vi "Measurement Parser.vi"(8 "error in (no error)":errorcluster, 10 "Data Array":dbl[](array[numeric]), 11 "Yokogawa WT2X0 in":refnum<class "Yokogawa WT2X0.lvclass">) -> (0 "error out":errorcluster, 2 "output cluster":T1, 3 "Yokogawa WT2X0 out":refnum<class "Yokogawa WT2X0.lvclass">)   [LabVIEW 2012, in "Universal Power Meter.lvlib" / "Yokogawa WT2X0.lvlib" / "Yokogawa WT2X0.lvclass"]
uses:
  Yokogawa WT2X0.lvclass
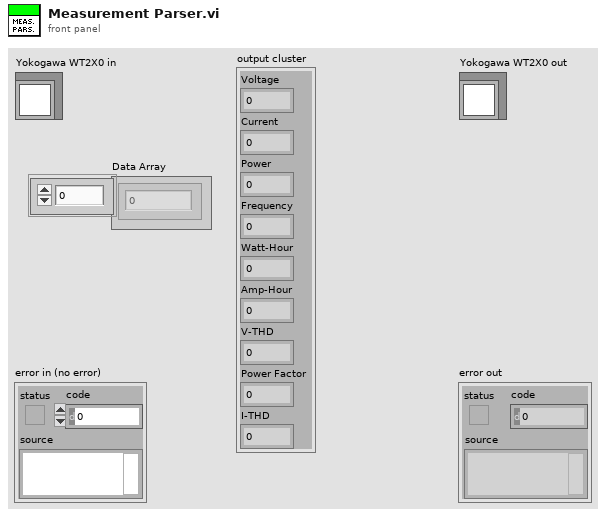
[diagram p1: front panel]
types:
  T1 = cluster{"Voltage":dbl, "Current":dbl, "Power":dbl, "Frequency":dbl, "Watt-Hour":dbl, "Amp-Hour":dbl, "V-THD":dbl, "Power Factor":dbl, "I-THD ":dbl}
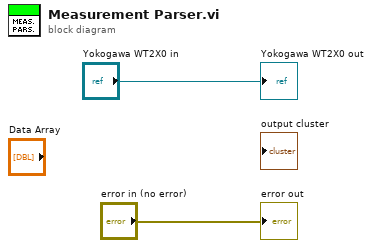
[diagram p0: block diagram]
diagram:
  "error out" <- "error in (no error)"
  "Yokogawa WT2X0 out" <- "Yokogawa WT2X0 in"
